vi "yellow--constant.vi"() -> (1 "Yellow":u32(colorbox))   [LabVIEW 2018]
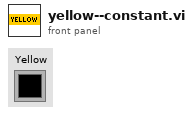
[diagram p1: front panel]
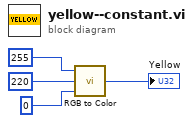
[diagram p0: block diagram]
diagram:
  n1 = call <vilib>:"RGB to Color.vi"("B"=u8 0, "G"=u8 220, "R"=u8 255) -> ("Color"=→"Yellow":u32)
